vi "GetResult.vi"(8 "error in (no error)":errorcluster, 11 "reference in":refnum<class "ProjectBuilder.lvclass">) -> (0 "error out":errorcluster, 2 "BrowerComponent":refnum<class "BrowerComponent.lvclass">, 3 "reference out":refnum<class "ProjectBuilder.lvclass">)   [LabVIEW 2015, in "ProjectBuilder.lvclass"]
uses:
  ProjectBuilder.lvclass
  BrowerComponent/BrowerComponent/BrowerComponent.lvclass
  ProjectBuilder.lvclass/ProjectBuilder.ctl
  Product/Interface/Part.lvclass
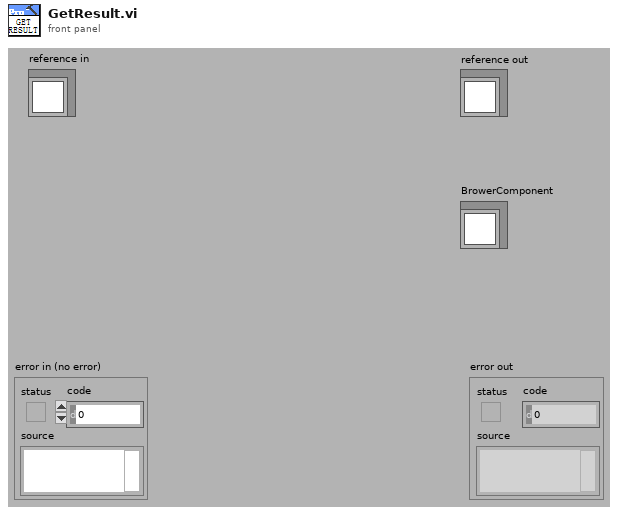
[diagram p1: front panel]
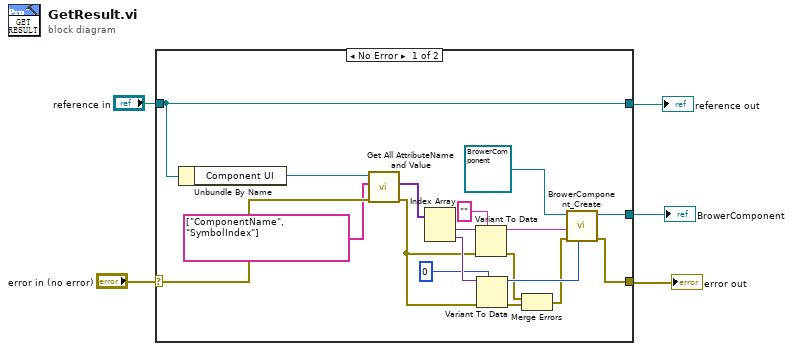
[diagram p0: block diagram]
diagram:
  n1 = case shown="No Error" "error in (no error)" {
    selector: "error in (no error)" -> [w21 w25]
    tunnel: [w7 w25] -> w4
    tunnel: [w23 w24] -> w2
    tunnel: "reference in" -> [w23 w24]
    tunnel: [w6 _] -> w1
    frame No Error {
      n2 = Unbundle By Name(w23) -> ("Component UI"=w22:refnum<class "Part.lvclass">)
      n3 = call "Get All AttributeName and Value.vi"("error in (no error)"=w21, "AttributeNames(\"\")"=string[] ["ComponentName", "SymbolIndex"], "Part in"=w22) -> ("error out"=w12:errorcluster, "AttributeValues"=w19:variant[])  [unwired: 6 in, 1 out]
      n4 = Index Array(array=w19) -> (element #1=w18:variant, element #2=w14:variant)  [unwired: 2 in]
      n5 = Variant To Data(error in=w12, type="", Variant=w18) -> (data=w16:string, error out=w9:errorcluster)
      n6 = Variant To Data(error in=w12, type=0 ("SymbolIndex"), Variant=w14) -> (data=w11:i32, error out=w10:errorcluster)
      n7 = Merge Errors(w9, w10) -> (w8:errorcluster)
      n8 = call "BrowerComponent_Create.vi"("SymbolIndex"=w11, "error in (no error)"=w8, "ComponentName"=w16, "reference in"=refnum<class "BrowerComponent.lvclass"> refnum ("BrowerComponent")) -> ("error out"=w7:errorcluster, "reference out"=w6:refnum<class "BrowerComponent.lvclass">)  [unwired: 6 in]
    }
    frame Error {
    }
  }
  "error out" <- w4
  "reference out" <- w2
  "BrowerComponent" <- w1
